vi "InsertStatusListBox.vi"(5 "In Line? (F)":bool, 6 "Clear Status (F)":bool, 8 "error in (no error)":errorcluster, 9 "Color (0-Black)":T1, 10 "Text in":string, 11 "Listbox":refnum<vi>) -> (0 "error out":errorcluster, 1 "Timestamp out":timestamp, 2 "Text out":string, 3 "reference out":refnum<vi>)   [LabVIEW 2020]
doc: "Inserts text into a specified listbox reference. A color can be selected but default is black. Best use for status listbox on a UI. Will automatically delete the first 1000 lines if list execeeds that amount."
uses:
  ListBoxColorText.ctl
  TD GetSemaphore Action--enum.ctl
  ListBoxReference.vi
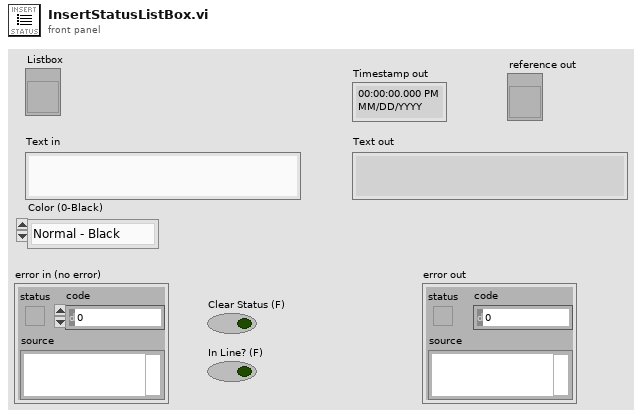
[diagram p1: front panel]
types:
  T1 = typedef "ListBoxColorText.ctl" = enum16{"Normal - Black", "Error - Red", "Sent - Blue", "Received - Green", "Debug - Magenta"}
  T2 = typedef "TD GetSemaphore Action--enum.ctl" = enum16{"Init", "Get", "NoOp"}
  T3 = typedef "Semaphore RefNum" = refnum<k1>
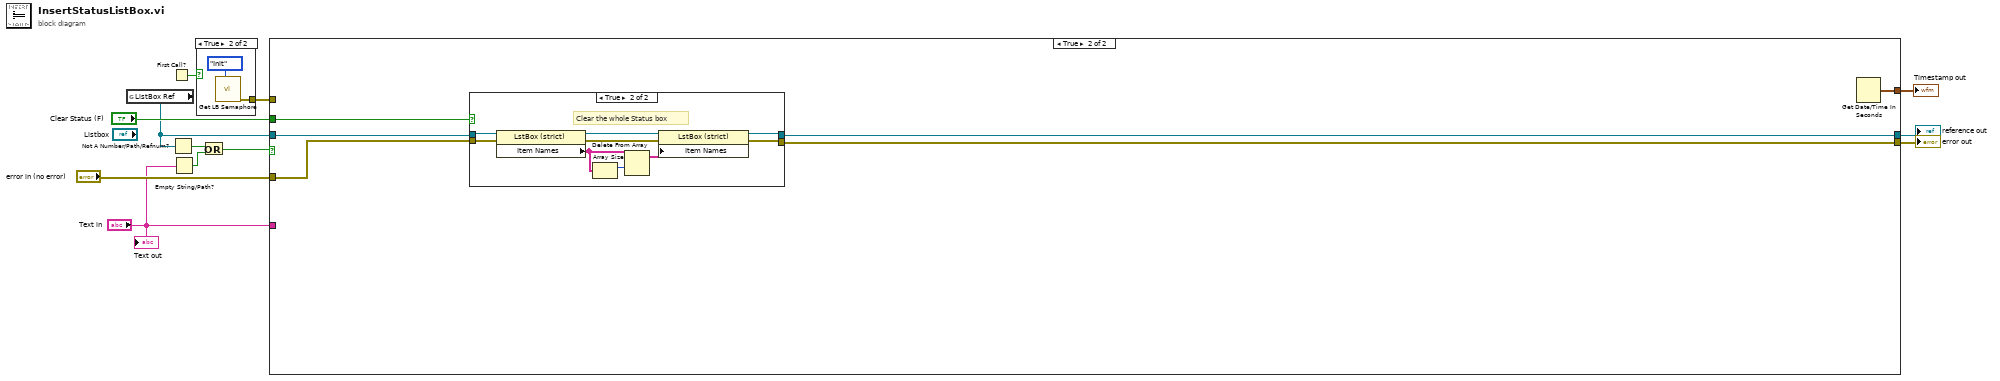
[diagram p0: block diagram]
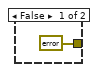
[diagram p2: hidden frame]
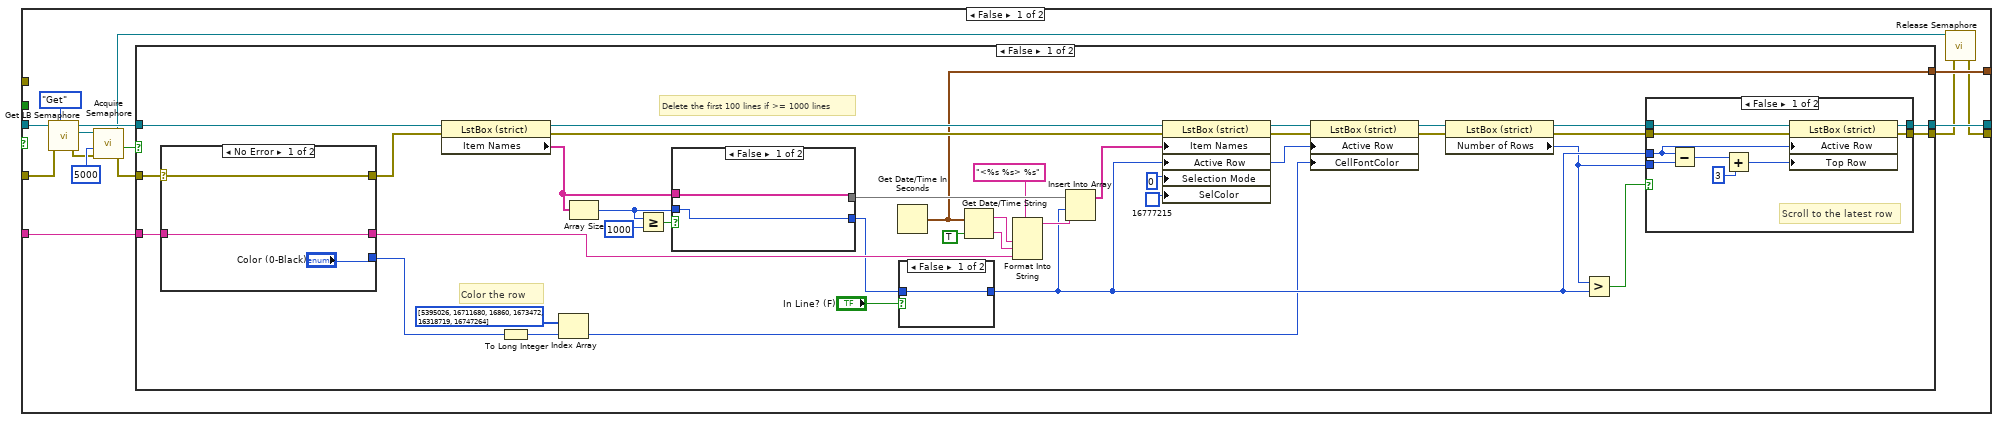
[diagram p3: hidden frame]
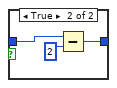
[diagram p4: hidden frame]
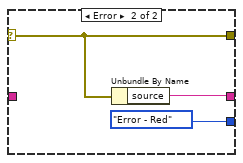
[diagram p6: hidden frame]
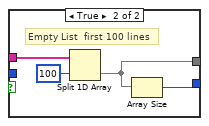
[diagram p7: hidden frame]
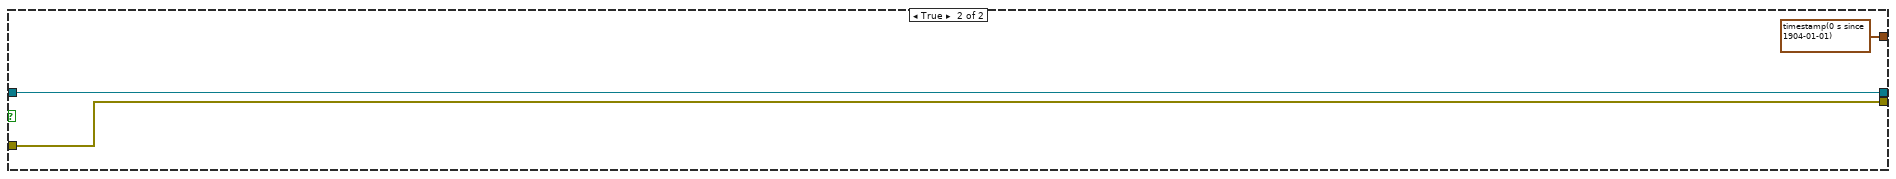
[diagram p8: hidden frame]
diagram:
  n1 = global read "ListBoxReference.vi" "ListBox Ref"() -> (w5:refnum<vi>)
  n2 = First Call?() -> (First Call?: T/F=w1:bool)
  n3 = Not A Number/Path/Refnum?(number/path/refnum=w5) -> (NaN/Path/Refnum?=w8:bool)
  n4 = Empty String/Path?(string/path="Text in") -> (empty?=w9:bool)
  n5 = case shown="True" w1 {
    tunnel: [errorcluster {"status"=FALSE, "code"=0, "source"=""} ("error out") w14] -> w2
    frame False {
    }
    frame True {
      n6 = call "Get LB Semaphore.vi"("action (Get)"=TD_GetSemaphore_Action--enum."Init") -> ("error out"=w14:errorcluster)  [unwired: 4 in, 3 out]
    }
  }
  n7 = Or(x=w8, y=w9) -> (x .or. y?=w7:bool)
  n8 = case shown="True" w7 {
    tunnel: [w21 w99] -> w12
    tunnel: [w29 w102] -> w11
    tunnel: w5 -> [w27 w104]
    tunnel: "error in (no error)" -> [w24 w103]
    tunnel: "Text in" -> [w30 _]
    tunnel: "Clear Status (F)" -> [_ w101]
    tunnel: [w28 w100] -> w3
    tunnel: w2 -> [_ _]
    frame False {
      n9 = call "Get LB Semaphore.vi"("action (Get)"=TD_GetSemaphore_Action--enum."Get", "error in"=w24, "LB reference in"=w27) -> ("error out"=w16:errorcluster, "semaphore out"=w18:T3, "LB reference out"=w26:refnum<vi>)  [unwired: 2 in, 1 out]
      n10 = call <vilib>:"Acquire Semaphore.vi"("error in (no error)"=w16, "ms timeout (-1)"=5000, "semaphore"=w18) -> ("error out"=w17:errorcluster, "timed out"=w22:bool, "semaphore out"=w19:T3)  [unwired: 2 in]
      n11 = case shown="False" w22 {
        tunnel: w30 -> [w51 _]
        tunnel: [w49 w98] -> w29
        tunnel: [w48 w97] -> w20
        tunnel: [w44 timestamp(0 s since 1904-01-01) ("seconds since 1Jan1904")] -> w28
        tunnel: w26 -> [w32 w98]
        tunnel: w17 -> [w31 w97]
        frame False {
          # "Color the row"
          # "Delete the first 100 lines if >= 1000 lines"
          n12 = case shown="No Error" w31 {
            selector: w31 -> [w86 w89]
            tunnel: [w84 w88] -> w57
            tunnel: [w86 w89] -> w53
            tunnel: ["Color (0-Black)" ListBoxColorText."Error - Red" ("Color (0-Black)")] -> w52
            tunnel: w51 -> [w84 _]
            frame No Error {
            }
            frame Error {
              n13 = Unbundle By Name(w89) -> ("source"=w88:string)
            }
          }
          n14 = property class="LstBox (strict)"(reference=w32, error in=w53) -> (reference out=w55:refnum<vi>, error out=w54:errorcluster, "Item Names"=w60:string[])
          n15 = To Long Integer(number=w52) -> (32bit integer=w43:i32)
          n16 = Index Array(array=u32[] [5395026, 16711680, 16860, 1673472, 16318719, 16747264] ("Color Cells"), index=w43) -> (element=w38:u32)
          n17 = Array Size(array=w60) -> (size(s)=w66:i32)
          n18 = Greater Or Equal?(x=w66, y=1000) -> (x >= y?=w67:bool)
          n19 = case shown="False" w67 {
            tunnel: w60 -> [w91 w94]
            tunnel: w66 -> [w90 _]
            tunnel: [w91 w92] -> w65
            tunnel: [w90 w95] -> w46
            frame False {
            }
            frame True {
              # "Empty List  first 100 lines"
              n20 = Split 1D Array(array=w94, index=100) -> (second subarray=w92:string[])  [unwired: 1 out]
              n21 = Array Size(array=w92) -> (size(s)=w95:i32)
            }
          }
          n22 = Get Date/Time In Seconds() -> (seconds since 1Jan1904=w44:timestamp)
          n23 = case shown="False" "In Line? (F)" {
            tunnel: w46 -> [w69 w71]
            tunnel: [w69 w72] -> w39
            frame False {
            }
            frame True {
              n24 = Subtract(x=w71, y=2) -> (x-y=w72:i32)
            }
          }
          n25 = Get Date/Time String(seconds (now)=w44, want seconds? (F)=TRUE) -> (date string=w64:string, time string=w63:string)  [unwired: 1 in]
          n26 = Format Into String(format string="<%s %s> %s", w64, w63, w57) -> (resulting string=w61:string)  [unwired: 2 in, 1 out]
          n27 = Insert Into Array(array=w65, index=w39, new element=w61) -> (w59:string[])
          n28 = property class="LstBox (strict)"(reference=w55, error in=w54, "Item Names"=w59, "Active Row"=w39, "Selection Mode"=0, "SelColor"=u32 16777215 ("Color Box")) -> (reference out=w40:refnum<vi>, error out=w41:errorcluster)
          n29 = property class="LstBox (strict)"(reference=w40, error in=w41, "Active Row"=w39, "CellFontColor"=w38) -> (reference out=w37:refnum<vi>, error out=w35:errorcluster)
          n30 = property class="LstBox (strict)"(reference=w37, error in=w35) -> (reference out=w36:refnum<vi>, error out=w34:errorcluster, "Number of Rows"=w33:u32)
          n31 = Greater?(x=w33, y=w39) -> (0:w47:bool)
          n32 = case shown="False" w47 {
            tunnel: w36 -> [w81 w83]
            tunnel: [w80 w83] -> w49
            tunnel: w34 -> [w79 w82]
            tunnel: [w78 w82] -> w48
            tunnel: w33 -> [w77 _]
            tunnel: w39 -> [w73 _]
            frame False {
              # "Scroll to the latest row"
              n33 = Subtract(x=w73, y=w77) -> (x-y=w75:u32)
              n34 = Add(x=w75, y=u32 3) -> (x+y=w74:u32)
              n35 = property class="LstBox (strict)"(reference=w81, error in=w79, "Active Row"=w73, "Top Row"=w74) -> (reference out=w80:refnum<vi>, error out=w78:errorcluster)
            }
            frame True {
            }
          }
        }
        frame True {
        }
      }
      n36 = call <vilib>:"Release Semaphore.vi"("error in (no error)"=w20, "semaphore"=w19) -> ("error out"=w21:errorcluster)  [unwired: 4 in, 1 out]
    }
    frame True {
      n37 = case shown="True" w101 {
        tunnel: w104 -> [w106 w109]
        tunnel: [w106 w108] -> w102
        tunnel: w103 -> [w105 w111]
        tunnel: [w105 w107] -> w99
        frame False {
        }
        frame True {
          # "Clear the whole Status box"
          n38 = property class="LstBox (strict)"(reference=w109, error in=w111) -> (reference out=w113:refnum<vi>, error out=w110:errorcluster, "Item Names"=w112:string[])
          n39 = Array Size(array=w112) -> (size(s)=w115:i32)
          n40 = Delete From Array(array=w112, length=w115) -> (array with subset deleted=w114:string[])  [unwired: 1 in, 1 out]
          n41 = property class="LstBox (strict)"(reference=w113, error in=w110, "Item Names"=w114) -> (reference out=w108:refnum<vi>, error out=w107:errorcluster)
        }
      }
      n42 = Get Date/Time In Seconds() -> (seconds since 1Jan1904=w100:timestamp)
    }
  }
  "error out" <- w12
  "reference out" <- w11
  "Timestamp out" <- w3
  "Text out" <- "Text in"
